vi "1.vi"() -> ()   [LabVIEW 2014]
panel:
  in  "stop":bool
  in  "YELLOW TIME 2":dbl
  in  "YELLOW TIME 2":dbl
  out "TIMER":dbl
  in  "GREEN TIME":dbl
  in  "YELLOW TIME":dbl
  in  "RED TIME":dbl
  out "GREEN":bool
  out "YELLOW":bool
  out "RED":bool
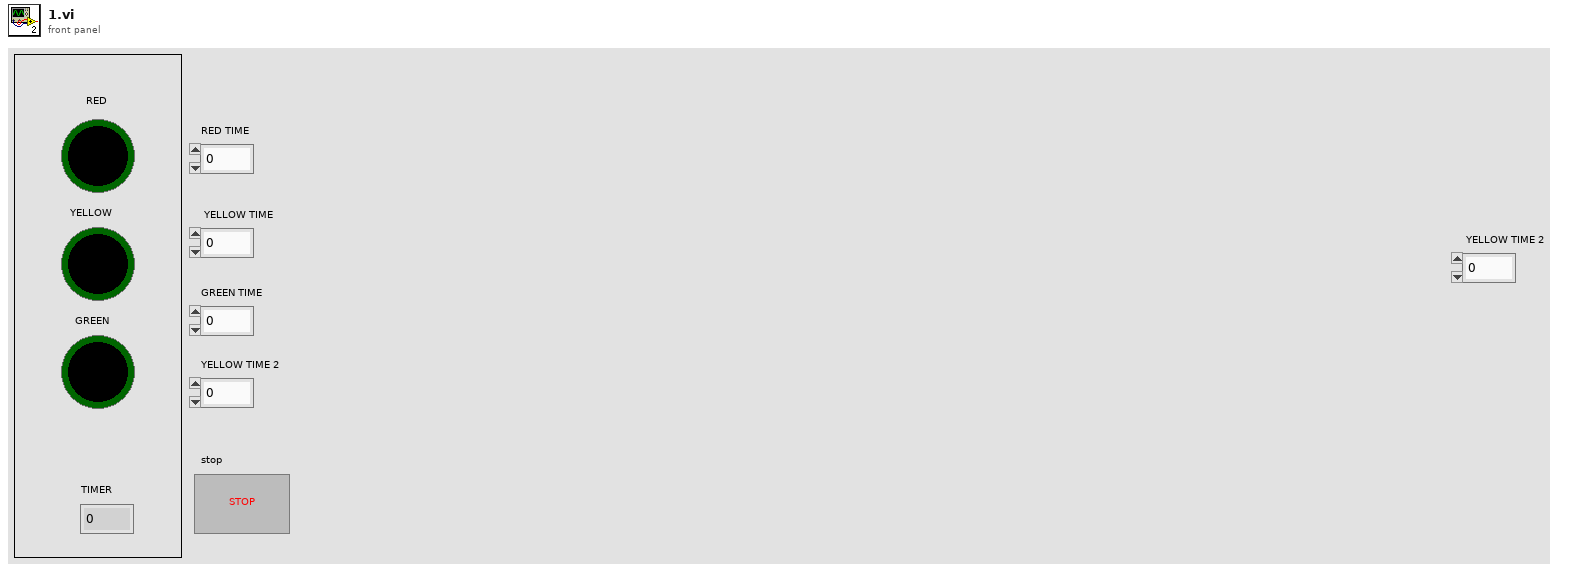
[diagram p1: front panel]
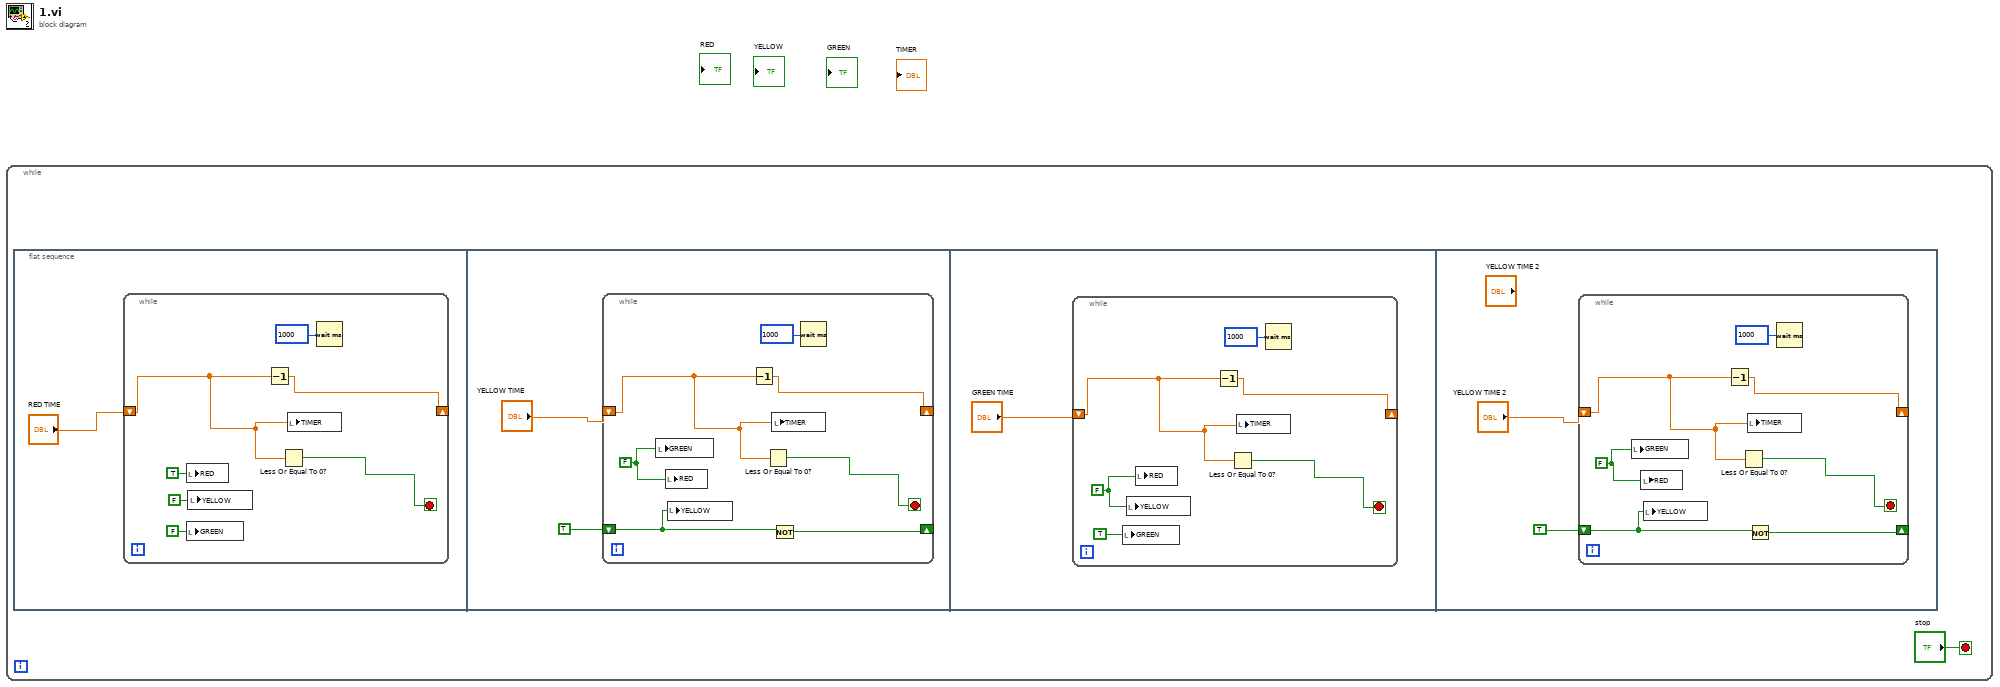
[diagram p0: block diagram]
diagram:
  n1 = while {
    stop <- "stop" stop-if-true
    n2 = flat-sequence {
      frame #0 {
        n3 = while {
          shift-right: [w8] -> _
          shift-left: "RED TIME" -> [w7]
          stop <- w6 stop-if-true
          n4 = local write "RED"(TRUE ("RED")) -> ()
          n5 = local write "GREEN"(FALSE ("GREEN")) -> ()
          n6 = local write "YELLOW"(FALSE ("YELLOW")) -> ()
          n7 = Decrement(x=w7) -> (x-1=w8:dbl)
          n8 = Less Or Equal To 0?(x=w7) -> (x <= 0?=w6:bool)
          n9 = local write "TIMER"(w7) -> ()
          n10 = Wait (ms)(milliseconds to wait=u32 1000) -> ()  [unwired: 1 out]
        }
      }
      frame #1 {
        n11 = while {
          shift-right: [w17] -> _
          shift-left: "YELLOW TIME" -> [w16]
          shift-right: [w12] -> _
          shift-left: TRUE -> [w13]
          stop <- w15 stop-if-true
          w14 = FALSE
          n12 = local write "GREEN"(w14) -> ()
          n13 = local write "RED"(w14) -> ()
          n14 = local write "YELLOW"(w13) -> ()
          n15 = Decrement(x=w16) -> (x-1=w17:dbl)
          n16 = Less Or Equal To 0?(x=w16) -> (x <= 0?=w15:bool)
          n17 = local write "TIMER"(w16) -> ()
          n18 = Not(x=w13) -> (.not. x?=w12:bool)
          n19 = Wait (ms)(milliseconds to wait=u32 1000) -> ()  [unwired: 1 out]
        }
      }
      frame #2 {
        n20 = while {
          shift-right: [w24] -> _
          shift-left: "GREEN TIME" -> [w23]
          stop <- w22 stop-if-true
          w20 = FALSE
          n21 = local write "GREEN"(TRUE) -> ()
          n22 = local write "YELLOW"(w20) -> ()
          n23 = local write "RED"(w20) -> ()
          n24 = Decrement(x=w23) -> (x-1=w24:dbl)
          n25 = Less Or Equal To 0?(x=w23) -> (x <= 0?=w22:bool)
          n26 = local write "TIMER"(w23) -> ()
          n27 = Wait (ms)(milliseconds to wait=u32 1000) -> ()  [unwired: 1 out]
        }
      }
      frame #3 {
        n28 = while {
          shift-right: [w33] -> _
          shift-left: "YELLOW TIME 2" -> [w32]
          shift-right: [w28] -> _
          shift-left: TRUE -> [w29]
          stop <- w31 stop-if-true
          w30 = FALSE
          n29 = local write "GREEN"(w30) -> ()
          n30 = local write "RED"(w30) -> ()
          n31 = local write "YELLOW"(w29) -> ()
          n32 = Decrement(x=w32) -> (x-1=w33:dbl)
          n33 = Less Or Equal To 0?(x=w32) -> (x <= 0?=w31:bool)
          n34 = local write "TIMER"(w32) -> ()
          n35 = Not(x=w29) -> (.not. x?=w28:bool)
          n36 = Wait (ms)(milliseconds to wait=u32 1000) -> ()  [unwired: 1 out]
        }
      }
    }
  }
